vi "FormIO.vi"() -> ()   [LabVIEW 2012]
uses:
  S7Ref.vi
panel:
  out "AI":T1 {"V    AI 7" format="%#.2g"; "V    AI 6" format="%#.2g"; "V    AI 5" format="%#.2g"; "V    AI 4" format="%#.2g"; "V    AI 3" format="%#.2g"; "V    AI 2" format="%#.2g"; "V    AI 1" format="%#.2g"; "V    AI 0" format="%#.2g"}
  in  "DQ 2":T2
  in  "DQ 3":T3
  out "DI 3":T3
  out "DI 4":T3
  out "DI 5":T3
  in  "DQ 4":T3
  in  "DQ 5":T3
  in  "DQ 6":T4
  in  "选项卡控件":enum32{"开关信号/操作", "传感器信号"}(tab)
  out "DI 2":T5
  out "DI 0":T6
  out "DI 1":T7
  in  "DQ 0":T8
  in  "DQ 1":T3
  # "输入上"
  # "输入下"
  # "输出上"
  # "输出下"
  # "输入正"
  # "输入反"
  # "输出正"
  # "输出反"
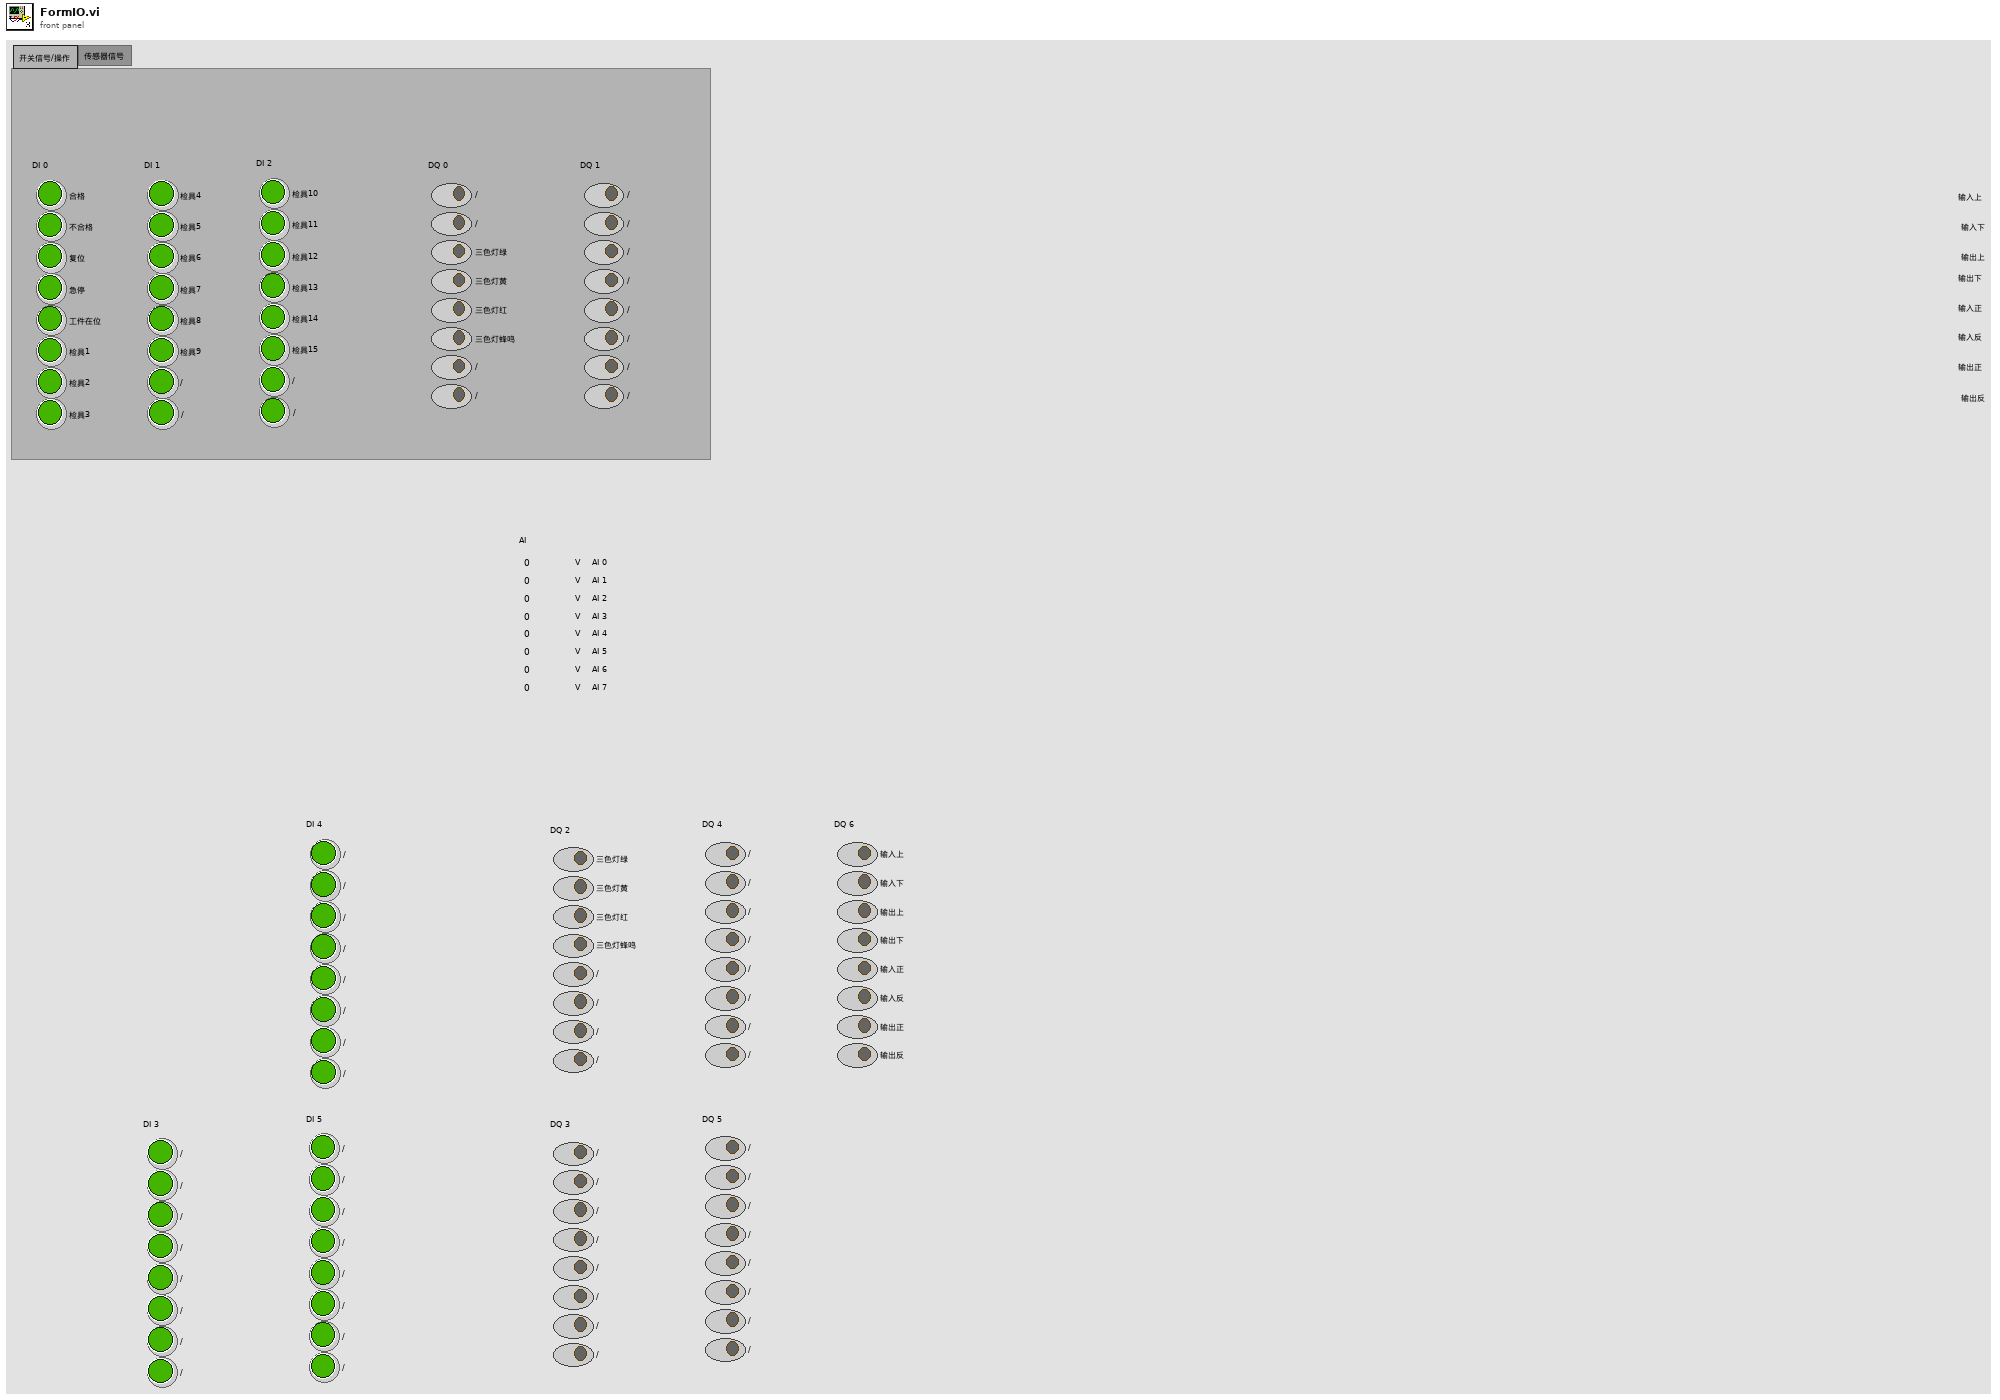
[diagram p1: front panel]
types:
  T1 = cluster{"V    AI 0":dbl, "V    AI 1":dbl, "V    AI 2":dbl, "V    AI 3":dbl, "V    AI 4":dbl, "V    AI 5":dbl, "V    AI 6":dbl, "V    AI 7":dbl}
  T2 = cluster{"三色灯绿":bool, "三色灯黄":bool, "三色灯红":bool, "三色灯蜂鸣":bool, "/":bool, "/":bool, "/":bool, "/":bool}
  T3 = cluster{"/":bool, "/":bool, "/":bool, "/":bool, "/":bool, "/":bool, "/":bool, "/":bool}
  T4 = cluster{"输入上":bool, "输入下":bool, "输出上":bool, "输出下":bool, "输入正":bool, "输入反":bool, "输出正":bool, "输出反":bool}
  T5 = cluster{"检具10":bool, "检具11":bool, "检具12":bool, "检具13":bool, "检具14":bool, "检具15":bool, "/":bool, "/":bool}
  T6 = cluster{"合格":bool, "不合格":bool, "复位":bool, "急停":bool, "工件在位":bool, "检具1":bool, "检具2":bool, "检具3":bool}
  T7 = cluster{"检具4":bool, "检具5":bool, "检具6":bool, "检具7":bool, "检具8":bool, "检具9":bool, "/":bool, "/":bool}
  T8 = cluster{"/":bool, "/":bool, "三色灯绿":bool, "三色灯黄":bool, "三色灯红":bool, "三色灯蜂鸣":bool, "/":bool, "/":bool}
  T9 = cluster{"输入移正脉冲":bool, "输入移反脉冲":bool, "输出移正脉冲":bool, "输出移反脉冲":bool, "控制器转速":bool, "/":bool, "控制器车速":bool, "/":bool}
  T10 = cluster{bool, bool, bool, bool, bool, bool, bool, bool}
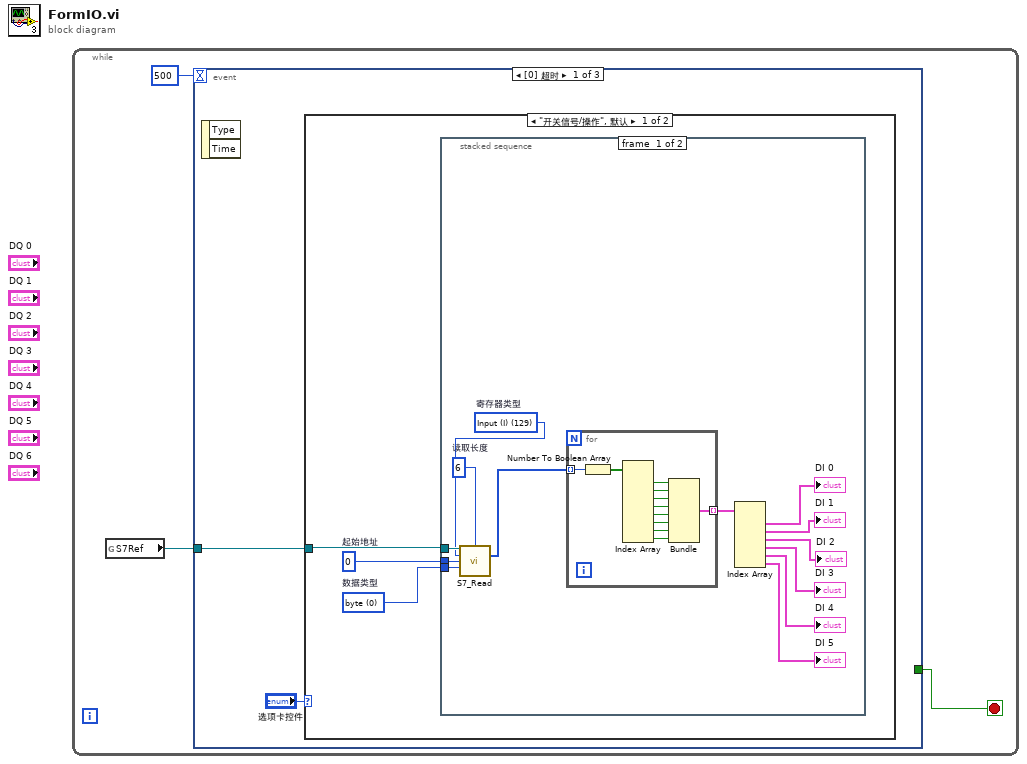
[diagram p0: block diagram]
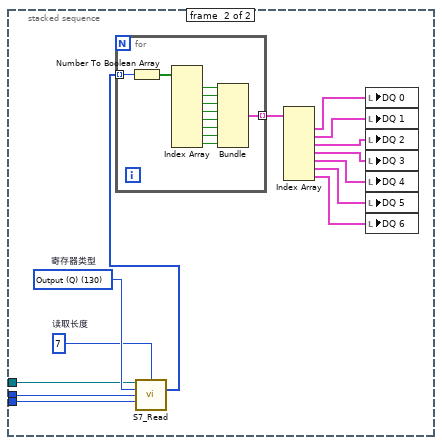
[diagram p2: hidden frame]
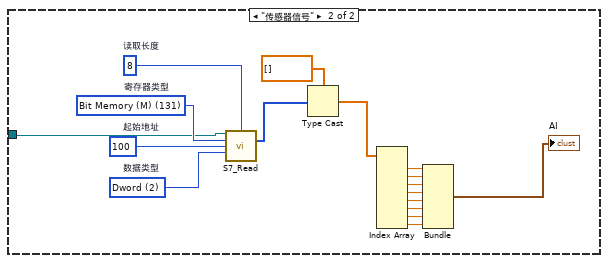
[diagram p3: hidden frame]
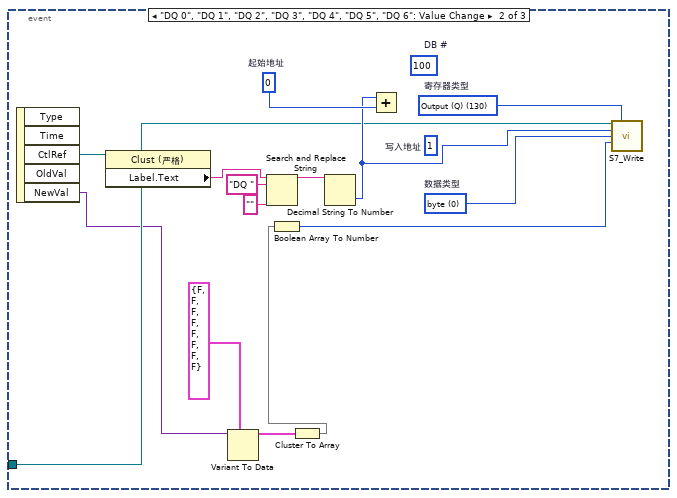
[diagram p4: hidden frame]
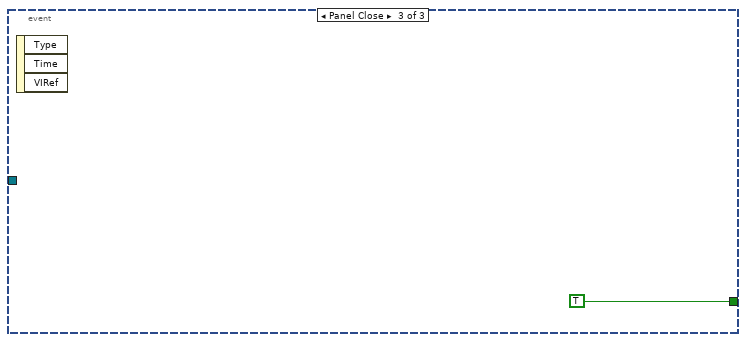
[diagram p5: hidden frame]
diagram:
  n1 = while {
    stop <- w3 stop-if-true
    n2 = global read "S7Ref.vi" "S7Ref"() -> (w1:refnum<k5>)
    n3 = event shown="[0] 超时" {
      selector: _ -> [_ _ _]
      dyn-events: _ -> [_ _ _]
      timeout: 500 -> [_ _ _]
      tunnel: [_ _ TRUE ("布尔")] -> w3
      tunnel: w1 -> [w4 w83 _]
      event Timeout {
        n4 = event-data() -> ()  [unwired: 1 in, 2 out]
        n5 = case shown="\"开关信号/操作\", 默认" "选项卡控件" {
          tunnel: w4 -> [w8 w69]
          frame "开关信号/操作", Default {
            w6 = u16 0 items=["byte", "word", "Dword"]  # 数据类型
            w7 = u32 0  # 起始地址
            n6 = stacked-sequence {
              tunnel: w8 -> [w21 w45]
              tunnel: w7 -> [w20 w44]
              tunnel: w6 -> [w19 w43]
              frame #0 {
                w10 = u16 6  # 读取长度
                w18 = u8 129 items=["I/O (P)"=128, "Input (I)"=129, "Output (Q)"=130, "Bit Memory (M)"=131, "Data (DB)"=132, "Instance Data (DI)"=133, "Local Data (L)"=134, "Predecessor Local Data (VL)"=135]  # 寄存器类型
                n7 = call "S7_Read.vi"("TCP"=w21, "读取长度"=w10, "寄存器类型"=w18, "起始地址"=w20, "数据类型"=w19) -> ("数据"=w17:u32[])  [unwired: 7 in, 3 out]
                n8 = for {
                  tunnel: w17 -> [w32] mode=indexing
                  tunnel: [w22] -> w16 mode=indexing
                  n9 = Number To Boolean Array(number=w32) -> (Boolean array=w31:bool[])
                  n10 = Index Array(array=w31) -> (element #1=w30:bool, element #2=w29:bool, element #3=w28:bool, element #4=w27:bool, element #5=w26:bool, element #6=w25:bool, element #7=w24:bool, element #8=w23:bool)  [unwired: 8 in]
                  n11 = Bundle(w30, w29, w28, w27, w26, w25, w24, w23) -> (w22:T10)  [unwired: 1 in]
                }
                n12 = Index Array(array=w16) -> (element #1=→"DI 0":T10, element #2=→"DI 1":T10, element #3=→"DI 2":T10, element #4=→"DI 3":T10, element #5=→"DI 4":T10, element #6=→"DI 5":T10)  [unwired: 6 in]
              }
              frame #1 {
                w33 = u16 7  # 读取长度
                w46 = u8 130 items=["I/O (P)"=128, "Input (I)"=129, "Output (Q)"=130, "Bit Memory (M)"=131, "Data (DB)"=132, "Instance Data (DI)"=133, "Local Data (L)"=134, "Predecessor Local Data (VL)"=135]  # 寄存器类型
                n13 = call "S7_Read.vi"("TCP"=w45, "读取长度"=w33, "寄存器类型"=w46, "起始地址"=w44, "数据类型"=w43) -> ("数据"=w41:u32[])  [unwired: 7 in, 3 out]
                n14 = for {
                  tunnel: w41 -> [w57] mode=indexing
                  tunnel: [w47] -> w42 mode=indexing
                  n15 = Number To Boolean Array(number=w57) -> (Boolean array=w56:bool[])
                  n16 = Index Array(array=w56) -> (element #1=w55:bool, element #2=w54:bool, element #3=w53:bool, element #4=w52:bool, element #5=w51:bool, element #6=w50:bool, element #7=w49:bool, element #8=w48:bool)  [unwired: 8 in]
                  n17 = Bundle(w55, w54, w53, w52, w51, w50, w49, w48) -> (w47:T10)  [unwired: 1 in]
                }
                n18 = Index Array(array=w42) -> (element #1=w40:T10, element #2=w39:T10, element #3=w38:T10, element #4=w37:T10, element #5=w36:T10, element #6=w35:T10, element #7=w34:T10)  [unwired: 7 in]
                n19 = local write "DQ 0"(w40) -> ()
                n20 = local write "DQ 1"(w39) -> ()
                n21 = local write "DQ 2"(w38) -> ()
                n22 = local write "DQ 3"(w37) -> ()
                n23 = local write "DQ 4"(w36) -> ()
                n24 = local write "DQ 5"(w35) -> ()
                n25 = local write "DQ 6"(w34) -> ()
              }
            }
          }
          frame "传感器信号" {
            w72 = u16 2 items=["byte", "word", "Dword"]  # 数据类型
            w73 = u32 100  # 起始地址
            w74 = u8 131 items=["I/O (P)"=128, "Input (I)"=129, "Output (Q)"=130, "Bit Memory (M)"=131, "Data (DB)"=132, "Instance Data (DI)"=133, "Local Data (L)"=134, "Predecessor Local Data (VL)"=135]  # 寄存器类型
            w71 = u16 8  # 读取长度
            n26 = call "S7_Read.vi"("TCP"=w69, "读取长度"=w71, "寄存器类型"=w74, "起始地址"=w73, "数据类型"=w72) -> ("数据"=w68:u32[])  [unwired: 7 in, 3 out]
            n27 = Type Cast(type=sgl[] [] ("添加的数组"), x=w68) -> (*(type *) &x=w59:sgl[])
            n28 = Index Array(array=w59) -> (element #1=w60:sgl, element #2=w61:sgl, element #3=w62:sgl, element #4=w63:sgl, element #5=w64:sgl, element #6=w65:sgl, element #7=w66:sgl, element #8=w67:sgl)  [unwired: 8 in]
            n29 = Bundle(w60, w61, w62, w63, w64, w65, w66, w67) -> (→"AI":cluster{sgl, sgl, sgl, sgl, sgl, sgl, sgl, sgl})  [unwired: 1 in]
          }
        }
      }
      event "DQ 0", "DQ 1", "DQ 2", "DQ 3", "DQ 4", "DQ 5", "DQ 6": Value Change {
        w86 = u32 0  # 起始地址
        w88 = u16 0 items=["byte", "word", "Dword"]  # 数据类型
        (unwired) u32 1  # 写入地址
        (unwired) u16 100  # DB #
        w89 = u8 130 items=["I/O (P)"=128, "Input (I)"=129, "Output (Q)"=130, "Bit Memory (M)"=131, "Data (DB)"=132, "Instance Data (DI)"=133, "Local Data (L)"=134, "Predecessor Local Data (VL)"=135]  # 寄存器类型
        n30 = event-data() -> ("CtlRef"=w85:refnum<vi>, "NewVal"=w81:variant)  [unwired: 1 in, 3 out]
        n31 = property class="Clust (严格)"(reference=w85) -> ("Label.Text"=w76:string)  [unwired: 1 in, 2 out]
        n32 = Variant To Data(type=T9 {"输入移正脉冲"=FALSE, "输入移反脉冲"=FALSE, "输出移正脉冲"=FALSE, "输出移反脉冲"=FALSE, "控制器转速"=FALSE, "/"=FALSE, "控制器车速"=FALSE, "/"=FALSE} ("DQ 0"), Variant=w81) -> (data=w80:T9)  [unwired: 1 in, 1 out]
        n33 = Search and Replace String(input string=w76, search string="DQ " ("搜索字符串"), replace string="" ("替换字符串(\"\")")) -> (result string=w75:string)  [unwired: 5 in, 3 out]
        n34 = Cluster To Array(cluster=w80) -> (array=w79:bool[])
        n35 = Boolean Array To Number ("布尔数组至数值转换")(Boolean array=w79) -> (number=w87:u8)
        n36 = Decimal String To Number(string=w75) -> (number=w84:i32)  [unwired: 2 in, 1 out]
        n37 = Add(x=w84, y=w86) -> ()  [unwired: 1 out]
        n38 = call "S7_Write.vi"("TCP"=w83, "寄存器类型"=w89, "写入地址"=w84, "数据类型"=w88, "写入数据"=w87) -> ()  [unwired: 8 in, 3 out]
      }
      event Panel Close {
        n39 = event-data() -> ()  [unwired: 1 in, 3 out]
      }
    }
  }
